vi "bkp1.vi"() -> ()   [LabVIEW 2020]
uses:
  <instrlib>/Agilent 34401/Public/Data/Read (Single Point).vi
  <instrlib>/Agilent E363X Series/Agilent E363X Series.lvlib
  <instrlib>/Agilent 34401/Agilent 34401.lvlib
panel:
  out "Courant":dbl
  in  "Tension":dbl
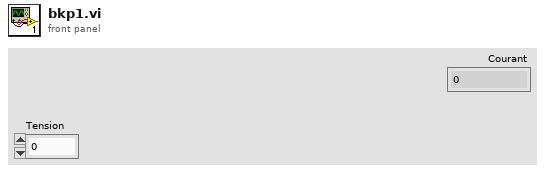
[diagram p1: front panel]
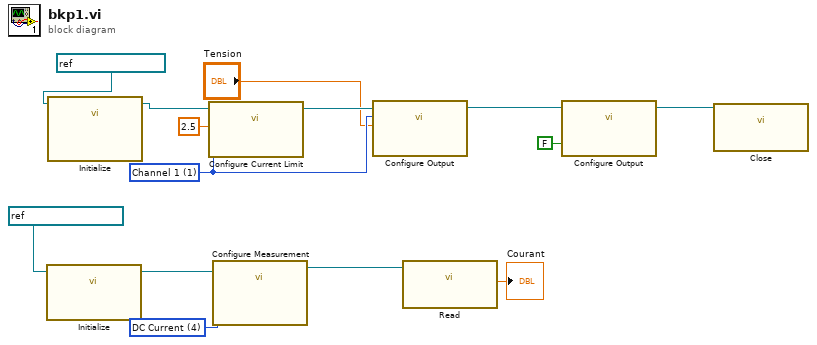
[diagram p0: block diagram]
diagram:
  w6 = u16 4 items=["DC Voltage", "AC Voltage", "2 - Wire Resistance", "4 - Wire Resistance", "DC Current", "AC Current", "Frequency", "Period", "Continuity", "Diode Checking", "VDC:VDC Ratio", "Temperature", "Capacitance"] ("Function (0: DC Voltage)")
  w11 = 1 items=["Channel 1"=1, "Channel 2"=2, "Channel 3"=3] ("Channel (1: Channel 1)")
  n1 = call <instrlib>:"Initialize.vi"("VISA resource name"=refnum<visa-resource-name> "GPIB0::22::INSTR") -> ("VISA resource name out"=w7:refnum<visa-resource-name>)  [unwired: 9 in, 1 out]
  n2 = call <instrlib>:"Initialize.vi"("VISA resource name"=refnum<visa-resource-name> "GPIB0::5::INSTR" ("VISA resource name out")) -> ("VISA resource name out"=w14:refnum<visa-resource-name>)  [unwired: 9 in, 1 out]
  n3 = call <instrlib>:"Configure Current Limit.vi"("Current Limit (0.0 A)"=2.5, "Channel (1: Channel 1)"=w11, "VISA resource name"=w14) -> ("VISA resource name out"=w12:refnum<visa-resource-name>)  [unwired: 7 in, 1 out]
  n4 = call <instrlib>:"Configure Measurement.vi"("Function (0: DC Voltage)"=w6, "VISA resource name"=w7) -> ("VISA resource name out"=w5:refnum<visa-resource-name>)  [unwired: 8 in, 1 out]
  n5 = call <instrlib>:"Configure Output.vi"("Voltage Level (0.0 V)"="Tension", "Channel (1: Channel 1)"=w11, "VISA resource name"=w12) -> ("VISA resource name out"=w3:refnum<visa-resource-name>)  [unwired: 7 in, 1 out]
  n6 = call-poly <instrlib>:"Read.vi"("VISA resource name"=w5) -> ("Measurement"=→"Courant":dbl)  [unwired: 8 in, 2 out]
  n7 = call <instrlib>:"Configure Output.vi"("Enable Output (T: Enable)"=FALSE, "VISA resource name"=w3) -> ("VISA resource name out"=w1:refnum<visa-resource-name>)  [unwired: 8 in, 1 out]
  n8 = call <instrlib>:"Close.vi"("VISA resource name"=w1) -> ()  [unwired: 10 in, 1 out]
